vi "Run Formatter.vi"(10 "Log Packet":T1, 11 "String Expression Format in":refnum<class "String Expression Format.lvclass">) -> (0 "error IO":errorcluster, 2 "Log Entry":string, 3 "String Expression Format out":refnum<class "String Expression Format.lvclass">)   [LabVIEW 2020, in "String Expression Format.lvclass"]
uses:
  <vilib>/gpm_packages/@cs/event-logger/Source/String Formats/String Expression Format/String Expression Format.lvclass
  <vilib>/gpm_packages/@cs/event-logger/Source/Composed Log/Types/Log Packet.ctl
  <vilib>/gpm_packages/@cs/event-logger/Source/Composed Log/Types/Log Level.ctl
  <vilib>/gpm_packages/@cs/event-logger/Source/String Formats/String Expression Format/String Expression Format.lvclass/String Expression Format.ctl
  <vilib>/gpm_packages/@cs/event-logger/Source/Composed Log/Composed Log.lvlib
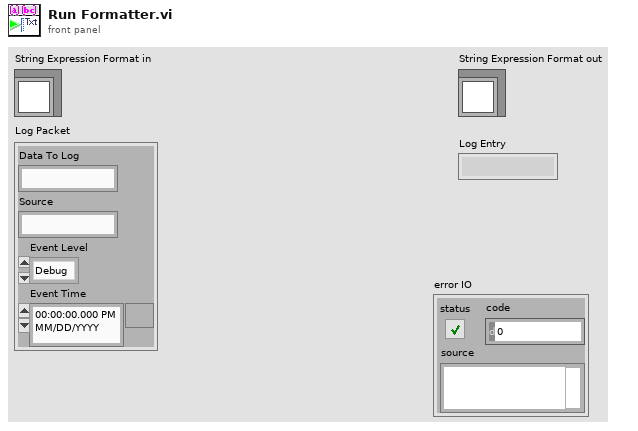
[diagram p1: front panel]
types:
  T1 = typedef "Composed Log.lvlib/Log Packet.ctl" = cluster{"Data To Log":string, "Source":string, "Event Level":T2, "Event Time":timestamp}
  T2 = typedef "Composed Log.lvlib/Log Level.ctl" = enum16{"Debug", "Info", "Warning", "Error", "Critical"}
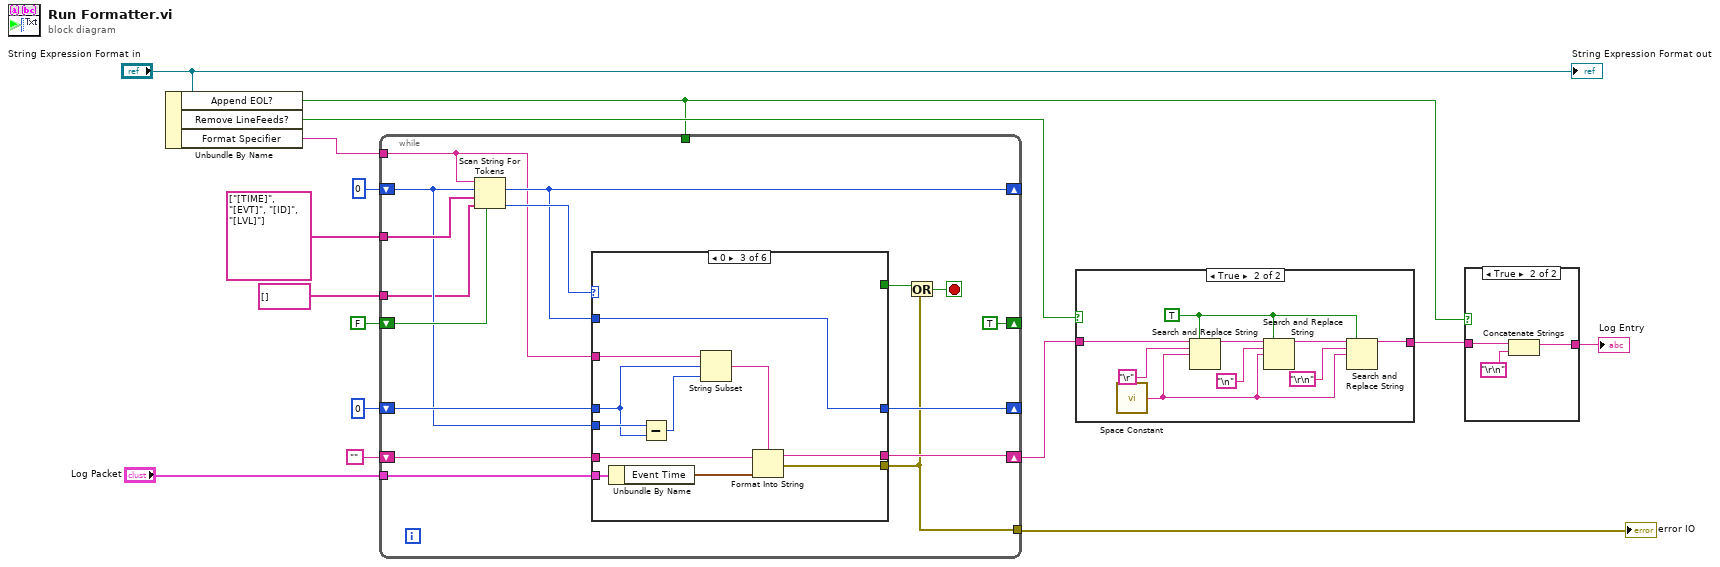
[diagram p0: block diagram]
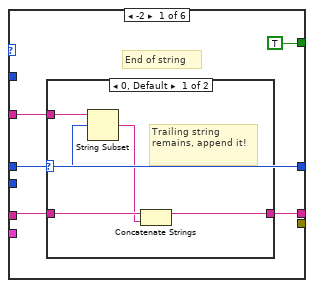
[diagram p4: hidden frame]
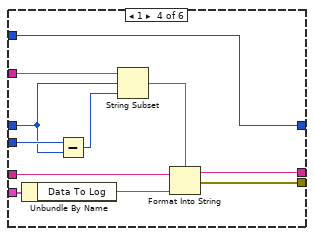
[diagram p7: hidden frame]
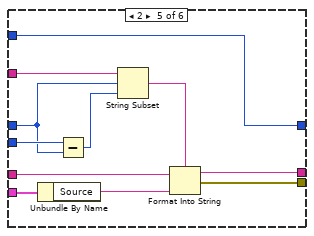
[diagram p8: hidden frame]
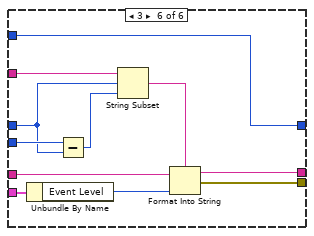
[diagram p9: hidden frame]
diagram:
  n1 = Unbundle By Name("String Expression Format in") -> ("Append EOL?"=w1:bool, "Remove LineFeeds?"=w2:bool, "Format Specifier"=w7:string)
  n2 = while {
    tunnel: string[] ["[TIME]", "[EVT]", "[ID]", "[LVL]"] ("appended array") -> [w31]
    shift-right: [w26] -> _
    shift-left: 0 ("offset past token") -> [w20]
    tunnel: "Log Packet" -> [w30]
    shift-right: [w27] -> _
    shift-left: 0 -> [w28]
    tunnel: string[] [] ("delimiters (\\s,\\t,\\r,\\n)") -> [w18]
    shift-right: [TRUE] -> _
    shift-left: FALSE -> [w25]
    shift-right: [w22] -> w4
    shift-left: "" -> [w23]
    tunnel: w7 -> [w19]
    tunnel: [w17] -> w5
    tunnel: w1 -> [_]
    stop <- w21 stop-if-true
    n3 = Scan String For Tokens(4:w25, 6:w18, 7:w31, 8:w20, 9:w19) -> (0:w29:i32, 2:w26:i32)  [unwired: 1 in, 2 out]
    n4 = case shown="0" w29 {
      tunnel: w30 -> [_ _ w55 w66 w77 w88]
      tunnel: w20 -> [_ w44 w50 w61 w72 w83]
      tunnel: w19 -> [w35 _ w53 w64 w75 w86]
      tunnel: w28 -> [w34 _ w49 w60 w71 w82]
      tunnel: [w34 w44 w51 w62 w73 w84] -> w27
      tunnel: w26 -> [_ _ w51 w62 w73 w84]
      tunnel: [_ _ w47 w58 w69 w80] -> w17
      tunnel: w23 -> [w36 w43 w46 w57 w68 w79]
      tunnel: [w33 w43 w45 w56 w67 w78] -> w22
      tunnel: [TRUE _ _ _ _ _] -> w16
      frame -2 {
        # "End of string"
        n5 = case shown="0, Default" w34 {
          selector: w34 -> [w37 _]
          tunnel: w36 -> [w41 w42]
          tunnel: w35 -> [w40 _]
          tunnel: [w39 w42] -> w33
          frame 0, Default {
            # "Trailing string remains, append it!"
            n6 = String Subset(string=w40, offset (0)=w37) -> (substring=w38:string)  [unwired: 1 in]
            n7 = Concatenate Strings(w41, w38) -> (w39:string)
          }
          frame -1 {
            # "Nothing at the end"
          }
        }
      }
      frame Default {
        # "not an operator"
      }
      frame 0 {
        n8 = Unbundle By Name(w55) -> ("Event Time"=w54:timestamp)
        n9 = Subtract(x=w50, y=w49) -> (x-y=w48:i32)
        n10 = String Subset(string=w53, offset (0)=w49, length (rest)=w48) -> (substring=w52:string)
        n11 = Format Into String(format string=w52, initial string=w46, w54) -> (resulting string=w45:string, error out=w47:errorcluster)  [unwired: 1 in]
      }
      frame 1 {
        n12 = Unbundle By Name(w66) -> ("Data To Log"=w65:string)
        n13 = Subtract(x=w61, y=w60) -> (x-y=w59:i32)
        n14 = String Subset(string=w64, offset (0)=w60, length (rest)=w59) -> (substring=w63:string)
        n15 = Format Into String(format string=w63, initial string=w57, w65) -> (resulting string=w56:string, error out=w58:errorcluster)  [unwired: 1 in]
      }
      frame 2 {
        n16 = Unbundle By Name(w77) -> ("Source"=w76:string)
        n17 = Subtract(x=w72, y=w71) -> (x-y=w70:i32)
        n18 = String Subset(string=w75, offset (0)=w71, length (rest)=w70) -> (substring=w74:string)
        n19 = Format Into String(format string=w74, initial string=w68, w76) -> (resulting string=w67:string, error out=w69:errorcluster)  [unwired: 1 in]
      }
      frame 3 {
        n20 = Unbundle By Name(w88) -> ("Event Level"=w87:T2)
        n21 = Subtract(x=w83, y=w82) -> (x-y=w81:i32)
        n22 = String Subset(string=w86, offset (0)=w82, length (rest)=w81) -> (substring=w85:string)
        n23 = Format Into String(format string=w85, initial string=w79, w87) -> (resulting string=w78:string, error out=w80:errorcluster)  [unwired: 1 in]
      }
    }
    n24 = Or(x=w16, y=w17) -> (x .or. y?=w21:bool)
  }
  "error IO" <- w5
  n25 = case shown="True" w2 {
    tunnel: w4 -> [w89 w96]
    tunnel: [w89 w94] -> w3
    frame False {
    }
    frame True {
      w95 = TRUE ("replace all? (F)")
      n26 = call <vilib>:"Space Constant.vi"() -> ("String"=w93:string)
      n27 = Search and Replace String(replace all?=w95, input string=w96, search string="\r", replace string=w93) -> (result string=w98:string)  [unwired: 4 in, 3 out]
      n28 = Search and Replace String(replace all?=w95, input string=w98, search string="\n", replace string=w93) -> (result string=w97:string)  [unwired: 4 in, 3 out]
      n29 = Search and Replace String(replace all?=w95, input string=w97, search string="\r\n", replace string=w93) -> (result string=w94:string)  [unwired: 4 in, 3 out]
    }
  }
  n30 = case shown="True" w1 {
    tunnel: w3 -> [w99 w101]
    tunnel: [w99 w100] -> w6
    frame False {
    }
    frame True {
      n31 = Concatenate Strings(w101, "\r\n") -> (w100:string)
    }
  }
  "Log Entry" <- w6
  "String Expression Format out" <- "String Expression Format in"
